vi "DBFill.vi"() -> ()   [LabVIEW 2015]
uses:
  lib/Snap7.lvlib
panel:
  out "?":string
  in  "FillChar":u8 format="%x"
  out "Running":bool
  out "Status":string="No Error"
  in  "DB Number":i32=1
  in  "?":bool
  in  "Slot":i32=2
  in  "Rack":i32
  in  "Address IP":string="192.168.1.12"
  # "DB Fill"
  # "WARNING !!!\nThis program will fill a DB Entirely"
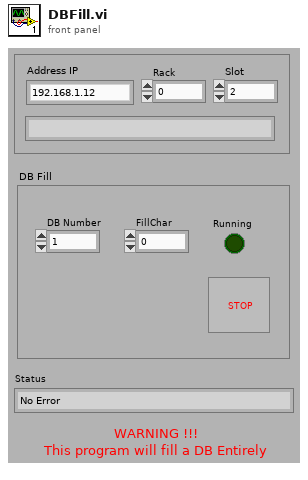
[diagram p1: front panel]
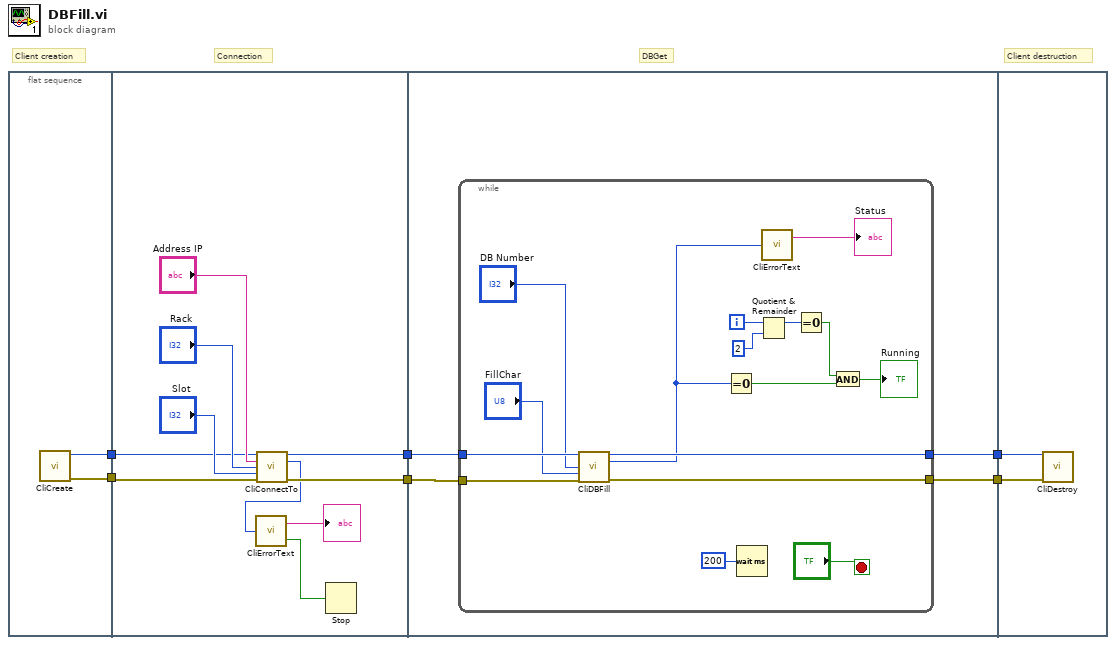
[diagram p0: block diagram]
diagram:
  # "Client destruction"
  # "DBGet"
  # "Connection"
  # "Client creation"
  n1 = flat-sequence {
    tunnel: [w8] -> w4
    tunnel: [w7] -> w3
    tunnel: [w18] -> w6
    tunnel: [w12] -> w5
    tunnel: w4 -> [w14]
    tunnel: w3 -> [w13]
    tunnel: w6 -> [w22]
    tunnel: w5 -> [w21]
    tunnel: [w20] -> w2
    tunnel: [w19] -> w1
    tunnel: w2 -> [w40]
    tunnel: w1 -> [w39]
    frame #0 {
      n2 = call "CliCreate.vi"() -> ("ref out"=w8:u64, "error out"=w7:errorcluster)  [unwired: 14 in]
    }
    frame #1 {
      n3 = call "CliConnectTo.vi"("ref in"=w14, "Address"="Address IP", "Rack"="Rack", "Slot"="Slot", "error in (no error)"=w13) -> ("ref out"=w12:u64, "Result"=w9:i32, "error out"=w18:errorcluster)  [unwired: 8 in]
      n4 = call "CliErrorText.vi"("ErrNo"=w9) -> ("Error"=w11:bool, "ErrMessage"=→"?":string)
      n5 = Stop(stop? (T)=w11) -> ()
    }
    frame #2 {
      n6 = while {
        tunnel: w22 -> [w29]
        tunnel: w21 -> [w30]
        tunnel: [w28] -> w19
        tunnel: [w27] -> w20
        i -> [w36]
        stop <- "?" stop-if-true
        n7 = call "CliDBFill.vi"("ref in"=w30, "DB Number"="DB Number", "FillChar"="FillChar", "error in (no error)"=w29) -> ("ref out"=w27:u64, "Result"=w24:i32, "error out"=w28:errorcluster)  [unwired: 9 in]
        n8 = Equal To 0?(x=w24) -> (x = 0?=w31:bool)
        n9 = Wait (ms)(milliseconds to wait=u32 200 ("Loop Delay (ms)")) -> ()  [unwired: 1 out]
        n10 = Quotient & Remainder(x=w36, y=2) -> (x-y*floor(x/y)=w34:i32)  [unwired: 1 out]
        n11 = call "CliErrorText.vi"("ErrNo"=w24) -> ("ErrMessage"=→"Status":string)  [unwired: 1 out]
        n12 = Equal To 0?(x=w34) -> (x = 0?=w33:bool)
        n13 = And(x=w33, y=w31) -> (x .and. y?=→"Running":bool)
      }
    }
    frame #3 {
      n14 = call "CliDestroy.vi"("ref in"=w40, "error in (no error)"=w39) -> ()  [unwired: 13 in, 1 out]
    }
  }
